vi "Main FPGA.vi"() -> ()   [LabVIEW 2014]
uses:
  <vilib>/rvi/Emulation/niFpgaGetClockAttributes.vi
  <vilib>/rvi/Emulation/niFpgaSctlEmulationGetInTimedLoop.vi
  <vilib>/rvi/Emulation/niFpgaEmulationReportErrorSimple.vi
  <vilib>/rvi/Emulation/niFpgaProcessEmulError.vi
  RT Watchdog/Watchdog Globals.vi
  <vilib>/rvi/eio/common/nirviEmuTemplateMethod_errors.vi
  <vilib>/rvi/Emulation/niFpgaCriticalErrorInLSC.vi
  <vilib>/rvi/interface/RandomDataEmulation/niFpgaRandomDataHandleErrors.vi
  <vilib>/eio/EIONode/EIONode.xnode
  <vilib>/rvi/DataTransferAndStorage/Container/XNode/niFpgaContainer.xnode
  <vilib>/rvi/interface/RandomDataEmulation/nirviRandomDataFpgaReadWriteTemplate.vi
panel:
  in  "PC CMD":bool
  out "AutoSwitch FB":bool
  in  "HVAC CMD":bool
  out "HVAC FB":bool
  out "CJC Output":T1
  out "TC Output":T2
  out "RT Safe?":bool
  out "Watchdog Safe?":bool
  in  "Gen East On/Off":bool
  in  "Gen West On/Off":bool
  out "Sensing":sgl[](array[numeric]) format="%2.1f"
  in  "CT Scales":sgl[](array[numeric])=[0.0, 0.0, 0.0, 0.0, 0.0, 0.0]
  in  "PV Bkr":bool
  in  "SSG Bkr":bool
  out "Fire Fault":bool
  out "Fire Alarm 2":bool
  out "Fire Alarm 1":bool
  out "SSG Bkr Aux":bool
  out "PV Bkr Aux":bool
  out "E-Stop Aux":bool
  in  "RT Safe":bool
  in  "Enable RT Watchdog":bool
  in  "Pet RT Watchdog":bool
  in  "RT Timeout Period (ticks)":u32=40000000 format="%.0p"
  in  "RT Reset on Watchdog Failure?":bool
  out "Time Since Last RT Pet":u32 format="%#.5p"
  # "Digital I/O"
  # "Watchdog"
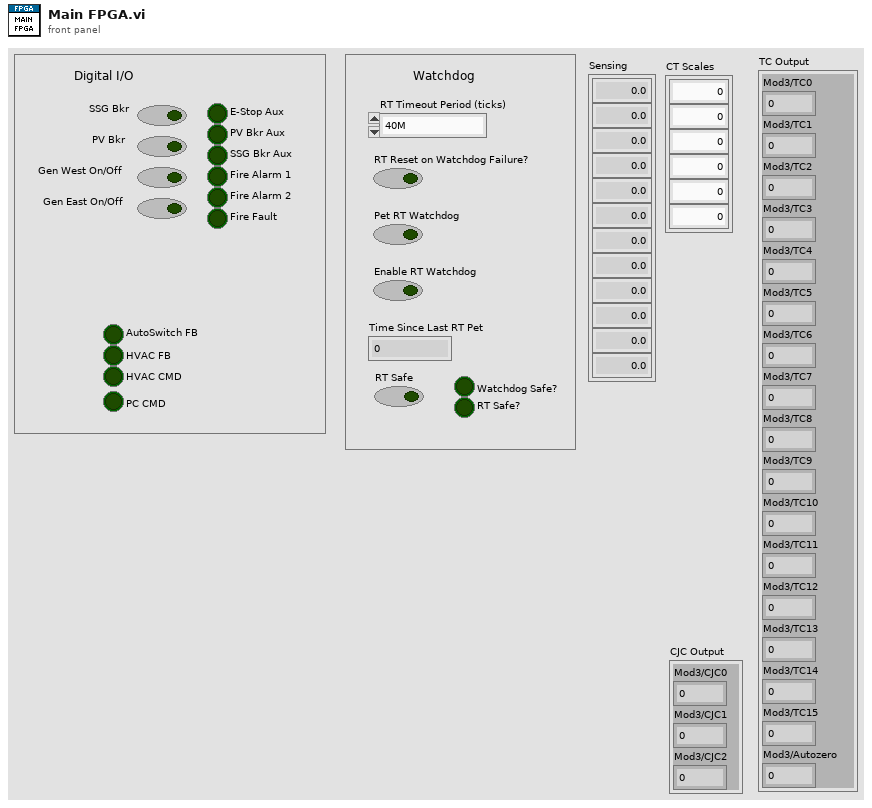
[diagram p1: front panel]
types:
  T1 = cluster{"Mod3/CJC0":fxp<+/-,24,-2>, "Mod3/CJC1":fxp<+/-,24,-2>, "Mod3/CJC2":fxp<+/-,24,-2>}
  T2 = cluster{"Mod3/TC0":fxp<+/-,24,-2>, "Mod3/TC1":fxp<+/-,24,-2>, "Mod3/TC2":fxp<+/-,24,-2>, "Mod3/TC3":fxp<+/-,24,-2>, "Mod3/TC4":fxp<+/-,24,-2>, "Mod3/TC5":fxp<+/-,24,-2>, "Mod3/TC6":fxp<+/-,24,-2>, "Mod3/TC7":fxp<+/-,24,-2>, "Mod3/TC8":fxp<+/-,24,-2>, "Mod3/TC9":fxp<+/-,24,-2>, "Mod3/TC10":fxp<+/-,24,-2>, "Mod3/TC11":fxp<+/-,24,-2>, "Mod3/TC12":fxp<+/-,24,-2>, "Mod3/TC13":fxp<+/-,24,-2>, "Mod3/TC14":fxp<+/-,24,-2>, "Mod3/TC15":fxp<+/-,24,-2>, "Mod3/Autozero":fxp<+/-,24,-2>}
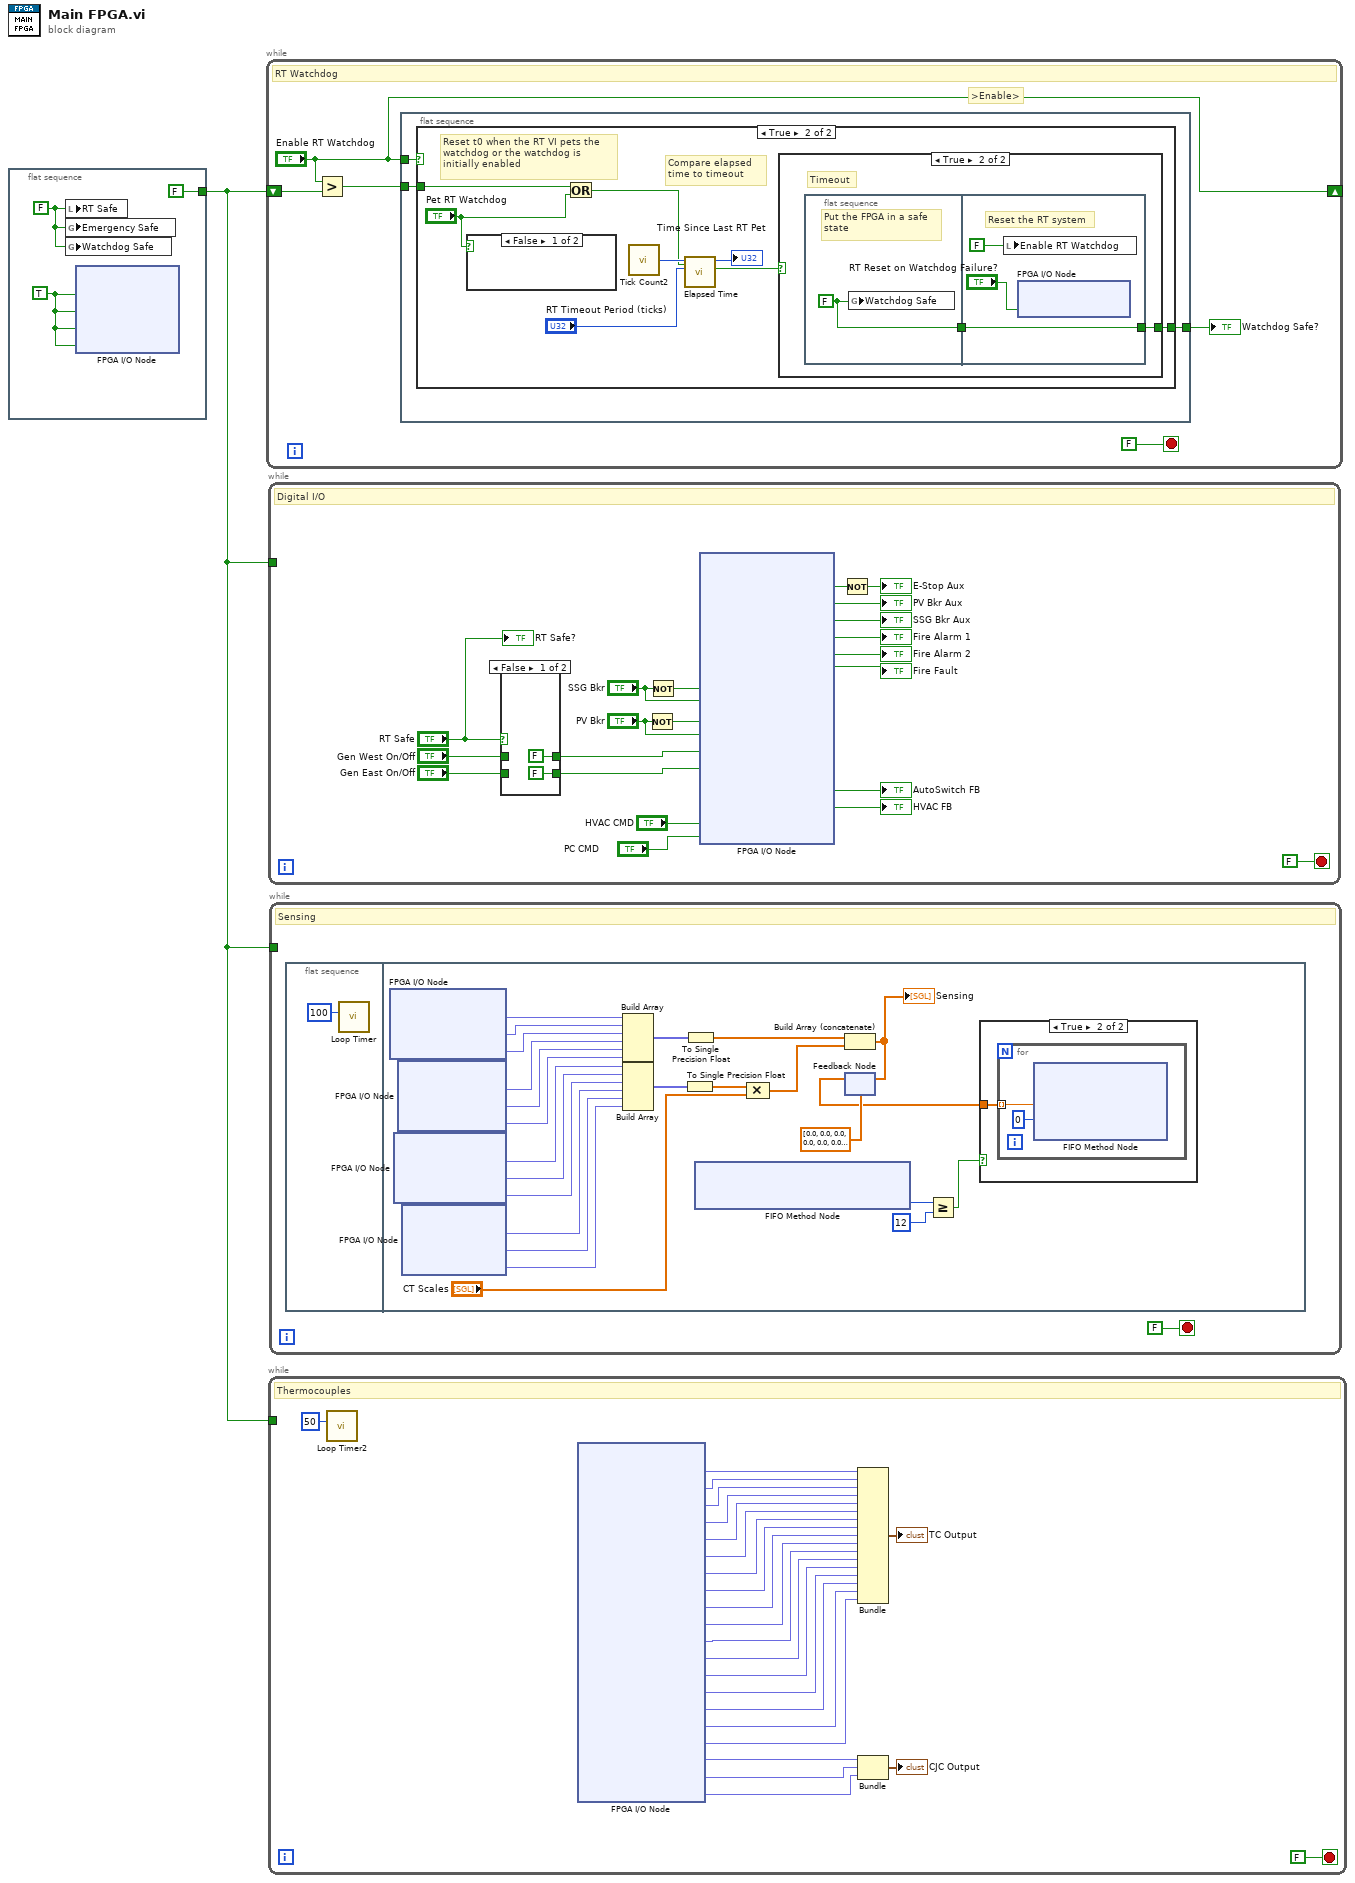
[diagram p0: block diagram]
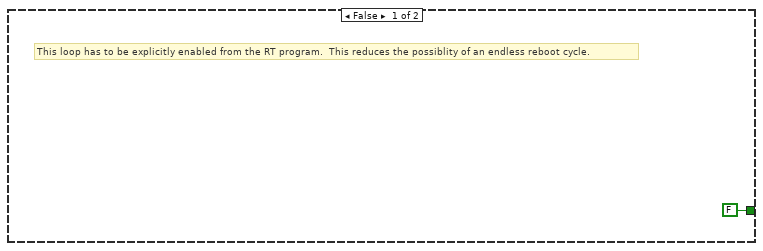
[diagram p3: hidden frame]
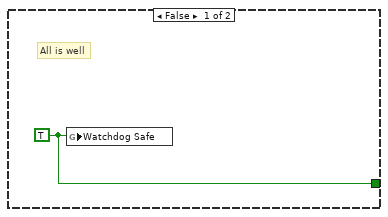
[diagram p4: hidden frame]
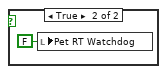
[diagram p5: hidden frame]
diagram:
  n1 = flat-sequence {
    tunnel: [FALSE ("Enable RT Watchdog")] -> w1
    frame #0 {
      w3 = TRUE ("Mod7/Start")
      w4 = FALSE ("RT Safe")
      n2 = local write "RT Safe"(w4) -> ()
      n3 = global write "Watchdog Globals.vi" "Emergency Safe"(w4) -> ()
      n4 = global write "Watchdog Globals.vi" "Watchdog Safe"(w4) -> ()
      n5 = xnode "FPGA I/O Node"("Mod5/Start"=w3, "Mod6/Start"=w3, "Mod7/Start"=w3, "Mod8/Start"=w3) -> ()  [unwired: 4 in, 4 out]
    }
  }
  n6 = while "RT Watchdog Loop" {
    shift-right: ["Enable RT Watchdog"] -> _
    shift-left: w1 -> [w9]
    stop <- FALSE stop-if-true
    # ">Enable>"
    # "RT Watchdog"
    n7 = Greater?(x="Enable RT Watchdog", y=w9) -> (0:w6:bool)
    n8 = flat-sequence {
      tunnel: "Enable RT Watchdog" -> [w12]
      tunnel: w6 -> [w11]
      tunnel: [w10] -> w5
      frame #0 {
        n9 = case shown="True" w12 {
          tunnel: w11 -> [_ w17]
          tunnel: [FALSE ("State Change") w14] -> w10
          frame False {
            # "This loop has to be explicitly enabled from the RT program.  This reduces the possiblity of an endless reboot cycle."
          }
          frame True {
            # "Compare elapsed time to timeout"
            # "Reset t0 when the RT VI pets the watchdog or the watchdog is initially enabled"
            n10 = case shown="False" "Pet RT Watchdog" {
              frame False {
              }
              frame True {
                n11 = local write "Pet RT Watchdog"(FALSE ("Pet RT Watchdog")) -> ()
              }
            }
            n12 = Or(x=w17, y="Pet RT Watchdog") -> (x .or. y?=w16:bool)
            n13 = call "Tick Count2"() -> ("Tick Count(Ticks)"=w20:u32)
            n14 = call "Elapsed Time.vi"("Reset"=w16, "Timeout Period"="RT Timeout Period (ticks)", "Current Time"=w20) -> ("Timeout"=w15:bool, "Elapsed Time"=→"Time Since Last RT Pet":u64)  [unwired: 7 in]
            n15 = case shown="True" w15 {
              tunnel: [w22 w23] -> w14
              frame False {
                w22 = TRUE ("State Change")
                # "All is well"
                n16 = global write "Watchdog Globals.vi" "Watchdog Safe"(w22) -> ()
              }
              frame True {
                # "Timeout"
                n17 = flat-sequence {
                  tunnel: [w25] -> w24
                  tunnel: w24 -> [w26]
                  tunnel: [w26] -> w23
                  frame #0 {
                    w25 = FALSE ("State Change")
                    # "Put the FPGA in a safe\nstate"
                    n18 = global write "Watchdog Globals.vi" "Watchdog Safe"(w25) -> ()
                  }
                  frame #1 {
                    # "Reset the RT system"
                    n19 = local write "Enable RT Watchdog"(FALSE ("Enable RT Watchdog")) -> ()
                    n20 = xnode "FPGA I/O Node"("System Reset"="RT Reset on Watchdog Failure?") -> ()  [unwired: 1 in, 1 out]
                  }
                }
              }
            }
          }
        }
      }
    }
    "Watchdog Safe?" <- w5
  }
  n21 = while "Digital I/O" {
    tunnel: w1 -> [_]
    stop <- FALSE stop-if-true
    # "Digital I/O"
    n22 = case shown="False" "RT Safe" {
      tunnel: "Gen West On/Off" -> [_ w53]
      tunnel: "Gen East On/Off" -> [_ w54]
      tunnel: [FALSE ("Gen East On/Off") w54] -> w43
      tunnel: [FALSE ("Gen West On/Off") w53] -> w42
      frame False {
      }
      frame True {
      }
    }
    n23 = Not(x="PV Bkr") -> (.not. x?=w39:bool)
    n24 = Not(x="SSG Bkr") -> (.not. x?=w40:bool)
    n25 = xnode "FPGA I/O Node"("SSG Bkr Open"=w40, "SSG Bkr Close"="SSG Bkr", "PV Bkr Open"=w39, "PV Bkr Close"="PV Bkr", "Gen West On/Off"=w42, "Gen East On/Off"=w43, "HVAC CMD"="HVAC CMD", "Rst Pwr Conv"="PC CMD") -> ("E-Stop Aux"=w35:bool, "PV Bkr Aux"=→"PV Bkr Aux":bool, "SSG Bkr Aux"=→"SSG Bkr Aux":bool, "Fire Alarm 1"=→"Fire Alarm 1":bool, "Fire Alarm 2"=→"Fire Alarm 2":bool, "Fire Fault"=→"Fire Fault":bool, "AutoSwitch FB"=→"AutoSwitch FB":bool, "HVAC FB"=→"HVAC FB":bool)  [unwired: 16 in, 16 out]
    n26 = Not(x=w35) -> (.not. x?=→"E-Stop Aux":bool)
    "RT Safe?" <- "RT Safe"
  }
  n27 = while {
    tunnel: w1 -> [_]
    stop <- FALSE stop-if-true
    # "Thermocouples"
    n28 = call "Loop Timer2"("Count(uSec)"=u32 50) -> ()  [unwired: 1 out]
    n29 = xnode "FPGA I/O Node"() -> ("Mod3/TC0"=w76:fxp<+/-,24,-2>, "Mod3/TC1"=w75:fxp<+/-,24,-2>, "Mod3/TC2"=w74:fxp<+/-,24,-2>, "Mod3/TC3"=w73:fxp<+/-,24,-2>, "Mod3/TC4"=w72:fxp<+/-,24,-2>, "Mod3/TC5"=w71:fxp<+/-,24,-2>, "Mod3/TC6"=w70:fxp<+/-,24,-2>, "Mod3/TC7"=w69:fxp<+/-,24,-2>, "Mod3/TC8"=w68:fxp<+/-,24,-2>, "Mod3/TC9"=w67:fxp<+/-,24,-2>, "Mod3/TC10"=w66:fxp<+/-,24,-2>, "Mod3/TC11"=w65:fxp<+/-,24,-2>, "Mod3/TC12"=w64:fxp<+/-,24,-2>, "Mod3/TC13"=w63:fxp<+/-,24,-2>, "Mod3/TC14"=w62:fxp<+/-,24,-2>, "Mod3/TC15"=w61:fxp<+/-,24,-2>, "Mod3/Autozero"=w60:fxp<+/-,24,-2>, "Mod3/CJC0"=w58:fxp<+/-,24,-2>, "Mod3/CJC1"=w57:fxp<+/-,24,-2>, "Mod3/CJC2"=w56:fxp<+/-,24,-2>)  [unwired: 20 in, 20 out]
    n30 = Bundle("Mod3/TC0"=w76, "Mod3/TC1"=w75, "Mod3/TC2"=w74, "Mod3/TC3"=w73, "Mod3/TC4"=w72, "Mod3/TC5"=w71, "Mod3/TC6"=w70, "Mod3/TC7"=w69, "Mod3/TC8"=w68, "Mod3/TC9"=w67, "Mod3/TC10"=w66, "Mod3/TC11"=w65, "Mod3/TC12"=w64, "Mod3/TC13"=w63, "Mod3/TC14"=w62, "Mod3/TC15"=w61, "Mod3/Autozero"=w60) -> (→"TC Output":T2)  [unwired: 1 in]
    n31 = Bundle("Mod3/CJC0"=w58, "Mod3/CJC1"=w57, "Mod3/CJC2"=w56) -> (→"CJC Output":T1)  [unwired: 1 in]
  }
  n32 = while {
    tunnel: w1 -> [_]
    stop <- FALSE stop-if-true
    # "Sensing"
    n33 = flat-sequence {
      frame #0 {
        n34 = call "Loop Timer"("Count(uSec)"=u32 100) -> ()  [unwired: 1 out]
      }
      frame #1 {
        n35 = xnode "FPGA I/O Node"() -> ("Input Vac (L1)"=w101:fxp<+/-,24,10>, "Input Vac (L2)"=w100:fxp<+/-,24,10>, "SSG Vac (L1)"=w99:fxp<+/-,24,10>)  [unwired: 3 in, 3 out]
        n36 = xnode "FPGA I/O Node"() -> ("Input Iac (L1)"=w92:fxp<+/-,24,5>, "Input Iac (L2)"=w91:fxp<+/-,24,5>, "SSG Iac (L1)"=w90:fxp<+/-,24,5>)  [unwired: 3 in, 3 out]
        n37 = xnode "FPGA I/O Node"() -> ("SSG Vac (L2)"=w98:fxp<+/-,24,10>, "PV Vac (L1)"=w97:fxp<+/-,24,10>, "PV Vac (L2)"=w96:fxp<+/-,24,10>)  [unwired: 3 in, 3 out]
        n38 = xnode "FPGA I/O Node"() -> ("SSG Iac (L2)"=w89:fxp<+/-,24,5>, "PV Iac (L1)"=w88:fxp<+/-,24,5>, "PV Iac (L2)"=w87:fxp<+/-,24,5>)  [unwired: 3 in, 3 out]
        n39 = Build Array(w101, w100, w99, w98, w97, w96) -> (w94:fxp<+/-,24,10>[])
        n40 = Build Array(w92, w91, w90, w89, w88, w87) -> (w93:fxp<+/-,24,5>[])
        n41 = To Single Precision Float(number=w93) -> (single precision float=w83:sgl[])
        n42 = To Single Precision Float(number=w94) -> (single precision float=w95:sgl[])
        n43 = xnode ("FIFO Method Node")() -> ("Number of Elements to Write"=w104:u32)  [unwired: 1 in, 1 out]
        n44 = Compound Arithmetic op=MULTIPLY(w83, "CT Scales") -> (w82:sgl[])
        n45 = Build Array (concatenate)(w95, w82) -> (w86:sgl[])
        "Sensing" <- w86
        n46 = feedback-in #1(w86) -> ()
        n47 = feedback #1(sgl[] [0.0, 0.0, 0.0, 0.0, 0.0, 0.0, 0.0, 0.0, 0.0, 0.0, 0.0, 0.0]) -> (w84:sgl[])
        n48 = Greater Or Equal?(x=w104, y=u32 12) -> (x >= y?=w102:bool)
        n49 = case shown="True" w102 {
          tunnel: w84 -> [_ w105]
          frame False {
          }
          frame True {
            n50 = for {
              tunnel: w105 -> [w107] mode=indexing
              n51 = xnode ("FIFO Method Node")("Element"=w107, "Timeout"=0) -> ()  [unwired: 1 in, 2 out]
            }
          }
        }
      }
    }
  }
